vi "Status-Set-Query SRER.vi"(8 "error in (no error)":errorcluster, 9 "sent to instrument":T1, 10 "function":bool, 11 "VISA resource name":refnum<visa-resource-name>) -> (0 "error out":errorcluster, 1 "read from instrument":T1, 3 "VISA resource name out":refnum<visa-resource-name>)   [LabVIEW 2016, in "Agilent 415X Series.lvlib"]
doc: "This VI sets or queries the bits in the instrument's IEEE-488.2 Service Request Enable Register."
uses:
  Agilent 415X Series.lvlib
panel:
  # "service request enable register"
  # "set\n\nquery"
  # "OPER       -        ESB     MAV   QUES      -       ME/ST EMER\n 128        64        32        16         8          4          2          1"
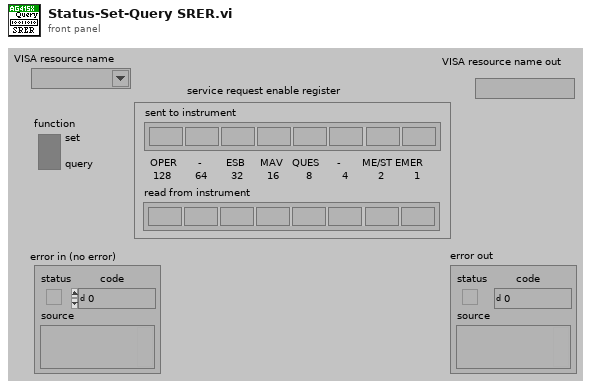
[diagram p1: front panel]
types:
  T1 = cluster{"   -":bool, "   -":bool, "   -":bool, "   -":bool, "   -":bool, "   -":bool, "   -":bool, "   -":bool}
  T2 = cluster{"[0]":bool, "[1]":bool, "[2]":bool, "[3]":bool, "[4]":bool, "[5]":bool, "[6]":bool, "[7]":bool}
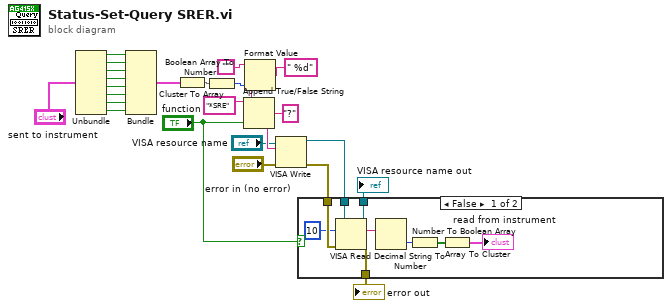
[diagram p0: block diagram]
diagram:
  n1 = Unbundle("sent to instrument") -> ("-"=w17:bool, "-"=w16:bool, "-"=w15:bool, "-"=w14:bool, "-"=w13:bool, "-"=w12:bool, "-"=w1:bool, "-"=w11:bool)
  n2 = Bundle("-"=w17, "-"=w16, "-"=w15, "-"=w14, "-"=w13, "-"=w12, "-"=w1, "-"=w11) -> (w9:T1)  [unwired: 1 in]
  n3 = Cluster To Array(cluster=w9) -> (array=w22:bool[])
  n4 = Boolean Array To Number(Boolean array=w22) -> (number=w21:u32)
  n5 = Format Value(string ("")="", format string=" %d", value (0)=w21) -> (output string=w24:string)
  n6 = Append True/False String(1:"function", 2:"?", 3:w24, 4:"*SRE") -> (0:w8:string)
  n7 = VISA Write(VISA resource name="VISA resource name", write buffer=w8, error in (no error)="error in (no error)") -> (VISA resource name out=w4:refnum<visa-resource-name>, error out=w5:errorcluster)  [unwired: 1 out]
  n8 = case shown="False" "function" {
    tunnel: w5 -> [w34 w35]
    tunnel: w4 -> [w29 w36]
    tunnel: [w28 w35] -> w3
    tunnel: [w27 w36] -> w2
    frame False {
      n9 = VISA Read(VISA resource name=w29, byte count=u32 10, error in (no error)=w34) -> (VISA resource name out=w27:refnum<visa-resource-name>, read buffer=w30:string, error out=w28:errorcluster)  [unwired: 1 out]
      n10 = Decimal String To Number(string=w30) -> (number=w33:i32)  [unwired: 2 in, 1 out]
      n11 = Number To Boolean Array(number=w33) -> (Boolean array=w32:bool[])
      n12 = Array To Cluster(array=w32) -> (cluster=→"read from instrument":T2)
    }
    frame True {
    }
  }
  "VISA resource name out" <- w2
  "error out" <- w3
